vi "About.vi"() -> ()   [LabVIEW 2014]
panel:
  out "已用(%):":dbl format="%#.2g"
  out "可用(M):":dbl
  in  "布尔":bool=TRUE
  # "XXXXXXXXXXXX系统软件3.0【标准版】"
  # "完成日期：2017.01.01"
  # "修订日期：2017.05.01"
  # "修订时间：12:30:21"
  # "版权：2017-2027 腾讯科技"
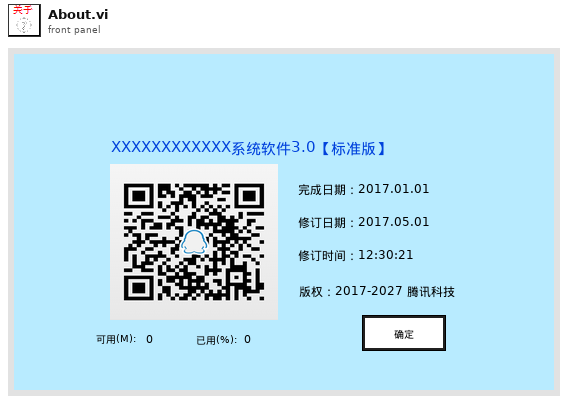
[diagram p1: front panel]
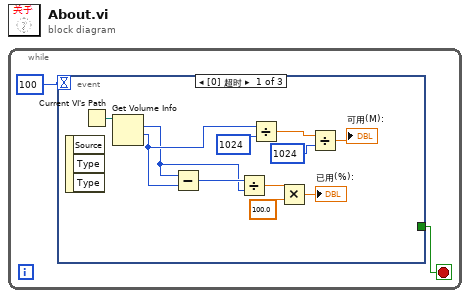
[diagram p0: block diagram]
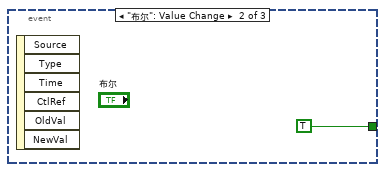
[diagram p2: hidden frame]
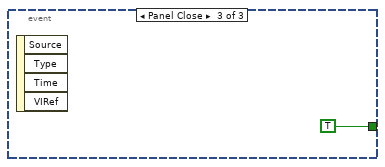
[diagram p3: hidden frame]
diagram:
  n1 = while {
    stop <- w2 stop-if-true
    n2 = event shown="[0] 超时" {
      selector: _ -> [_ _ _]
      dyn-events: _ -> [_ _ _]
      timeout: u32 100 ("等待时间（毫秒）") -> [_ _ _]
      tunnel: [_ TRUE TRUE] -> w2
      event Timeout {
        n3 = event-data() -> ()  [unwired: 1 in, 3 out]
        n4 = Current VI's Path() -> (path=w10:path)
        n5 = Get Volume Info(11:w10) -> (1:w4:i64, 2:w3:i64)  [unwired: 1 in, 4 out]
        n6 = Subtract(x=w3, y=w4) -> (x-y=w9:i64)
        n7 = Divide(x=w9, y=w3) -> (x/y=w11:dbl)
        n8 = Divide(x=w4, y=i64 1024) -> (x/y=w6:dbl)
        n9 = Multiply(x=w11, y=100.0) -> (x*y=→"已用(%):":dbl)
        n10 = Divide(x=w6, y=i64 1024) -> (x/y=→"可用(M):":dbl)
      }
      event "布尔": Value Change {
        n11 = event-data() -> ()  [unwired: 1 in, 6 out]
      }
      event Panel Close {
        n12 = event-data() -> ()  [unwired: 1 in, 4 out]
      }
    }
  }
